vi "LVCAM Create Nest.vi"(9 "Alias":string, 10 "Nest Actor":refnum<class "LVCAM.lvclass">, 11 "Self Actor in":refnum<class "Self Actor.lvclass">) -> (0 "error out":errorcluster, 3 "Self Actor out":refnum<class "Self Actor.lvclass">)   [LabVIEW 2021, in "LVCAM.lvlib" / "Self Actor.lvclass"]
uses:
  Self Actor.lvclass
  C:/PPLs/LabVIEW-Composed-Actor-Model-LVCAM/LabVIEW-Composed-Actor-Model-LVCAM/LVCAM/LVCAM/LVCAM/LVCAM.lvclass
  LVCAM/LVCAM.lvclass
  Self Actor.lvclass/Self Actor.ctl
  LVCAM/Msg Loop.vi
  Msg Q/Msg Q.lvclass
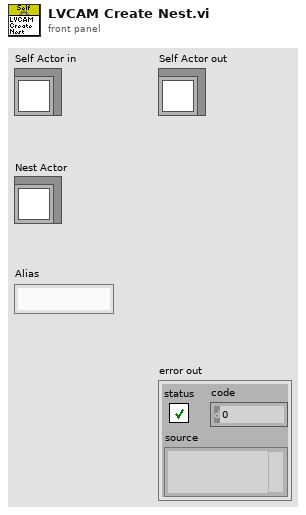
[diagram p1: front panel]
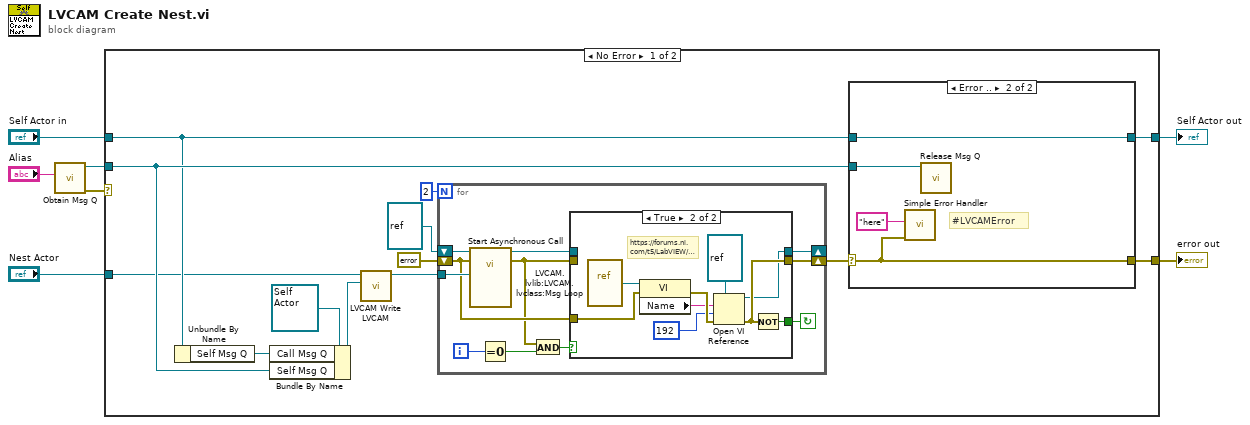
[diagram p0: block diagram]
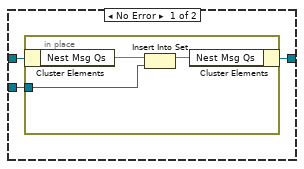
[diagram p2: hidden frame]
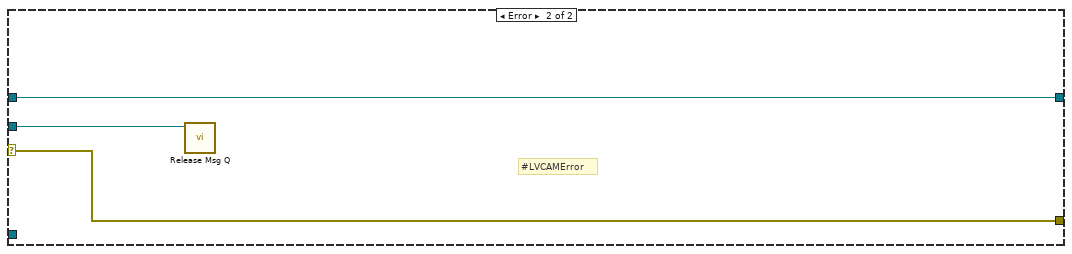
[diagram p4: hidden frame]
diagram:
  n1 = call "Obtain Msg Q.vi"("Alias"="Alias") -> ("error out"=w1:errorcluster, "Msg Queue out"=w3:refnum<class "Msg Q.lvclass">)  [unwired: 9 in]
  n2 = case shown="No Error" w1 {
    selector: w1 -> [_ w55]
    tunnel: [w20 w54] -> w6
    tunnel: [w14 w55] -> w5
    tunnel: "Nest Actor" -> [w8 _]
    tunnel: w3 -> [w10 w53]
    tunnel: "Self Actor in" -> [w9 w54]
    frame No Error {
      n3 = Unbundle By Name(w9) -> ("Self Msg Q"=w11:refnum<class "Msg Q.lvclass">)
      n4 = Bundle By Name(cluster=refnum<class "Self Actor.lvclass"> refnum ("Self Actor in"), "Call Msg Q"=w11, "Self Msg Q"=w10) -> (w12:refnum<class "Self Actor.lvclass">)
      n5 = call-dynamic "LVCAM Write LVCAM.vi"("LVCAM"=w12, "LVCAM Write LVCAM in"=w8) -> ("LVCAM Write LVCAM out"=w15:refnum<class "LVCAM.lvclass">)  [unwired: 9 in]
      n6 = for {
        N: 2 -> [_]
        tunnel: w15 -> [w41]
        shift-right: [w32] -> w19
        shift-left: errorcluster {"status"=FALSE, "code"=0, "source"=""} ("error out") -> [w35]
        shift-right: [w38] -> _
        shift-left: refnum<vi> refnum ("type specifier VI Refnum (for type only)") -> [w31]
        i -> [w40]
        stop <- w34 continue-if-true
        n7 = call-by-ref "Start Asynchronous Call"(reference=w31, error in=w35, "LVCAM in"=w41) -> (reference out=w37:refnum<vi>, error out=w33:errorcluster)  [unwired: 11 in]
        n8 = Equal To 0?(x=w40) -> (x = 0?=w39:bool)
        n9 = And(x=w33, y=w39) -> (x .and. y?=w36:bool)
        n10 = case shown="True" w36 {
          tunnel: [w42 w47] -> w38
          tunnel: w37 -> [w42 _]
          tunnel: w35 -> [_ w51]
          tunnel: w33 -> [w43 _]
          tunnel: [_ w52] -> w34
          tunnel: [w43 w48] -> w32
          frame False {
          }
          frame True {
            # "https://forums.ni.com/t5/LabVIEW/Static-VI-Reference/m-p/3334014#M978333"
            n11 = vi-ref "LVCAM.lvlib:LVCAM.lvclass:Msg Loop.vi"() -> (w45:refnum<vi>)
            n12 = property class="VI"(reference=w45, error in=w51) -> (error out=w50:errorcluster, "Name"=w49:string)  [unwired: 1 out]
            n13 = Open VI Reference(type specifier VI Refnum (for type only)=refnum<vi> refnum, vi path=w49, options=192 ("options: Multiple Clones,\n  Fire & Forget"), error in (no error)=w50) -> (vi reference=w47:refnum<vi>, error out=w48:errorcluster)  [unwired: 2 in]
            n14 = Not(x=w48) -> (.not. x?=w52:bool)
          }
        }
      }
      n15 = case shown="Error .." w19 {
        selector: w19 -> [_ w28]
        tunnel: w9 -> [w23 w30]
        tunnel: [w22 w30] -> w20
        tunnel: w10 -> [w21 w29]
        tunnel: [_ w28] -> w14
        frame No Error {
          n16 = in-place {
            in-place-border: w21 -> [w24]
            n17 = in-place-cluster #1(w23) -> ("Nest Msg Qs"=w26:set{refnum<class "Msg Q.lvclass">})
            n18 = Insert Into Set(10:w24, 11:w26) -> (3:w25:set{refnum<class "Msg Q.lvclass">})  [unwired: 1 out]
            n19 = in-place-cluster #1("Nest Msg Qs"=w25) -> (w22:refnum<class "Self Actor.lvclass">)
          }
        }
        frame Error {
          # "#LVCAMError"
          n20 = call <vilib>:"Simple Error Handler.vi"("error source (\" \")"="here" ("error source (\" \")"), "error in (no error)"=w28) -> ()  [unwired: 3 in, 5 out]
          n21 = call "Release Msg Q.vi"("Msg Queue in"=w29) -> ()  [unwired: 9 in, 2 out]
        }
      }
    }
    frame Error {
      # "#LVCAMError"
      n22 = call "Release Msg Q.vi"("Msg Queue in"=w53) -> ()  [unwired: 9 in, 2 out]
    }
  }
  "error out" <- w5
  "Self Actor out" <- w6
